vi "Error.set.vi"(8 "error in (no error)":errorcluster, 11 "ErrorDaemon in":refnum<class "ErrorDaemon.lvclass">) -> (0 "error out":errorcluster, 3 "ErrorDaemon out":refnum<class "ErrorDaemon.lvclass">)   [LabVIEW 2020, in "ErrorDaemon.lvclass"]
uses:
  ErrorDaemon.lvclass
  ErrorDaemon.lvclass/ErrorDaemon.ctl
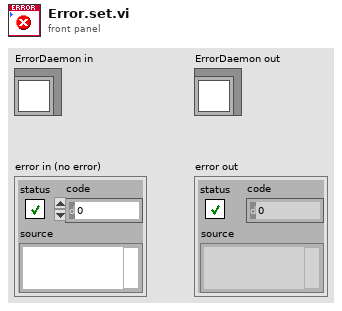
[diagram p1: front panel]
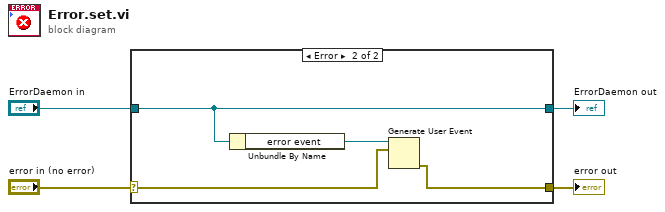
[diagram p0: block diagram]
diagram:
  n1 = case shown="Error" "error in (no error)" {
    selector: "error in (no error)" -> [w5 w8]
    tunnel: [w5 w7] -> w3
    tunnel: [w6 w10] -> w1
    tunnel: "ErrorDaemon in" -> [w6 w10]
    frame No Error {
    }
    frame Error {
      n2 = Unbundle By Name(w10) -> ("error event"=w9:refnum<user-event>)
      n3 = Generate User Event(user event=w9, event data cluster=w8) -> (error out=w7:errorcluster)  [unwired: 2 in, 1 out]
    }
  }
  "error out" <- w3
  "ErrorDaemon out" <- w1
